vi "post-4616-1160681073.vi"(3 "New angle":dbl format="%.2f", 4 "Previous angle":dbl format="%.2f", 5 "Position % (50)":dbl=50.0 format="%.2f", 6 "Width":dbl format="%.2f") -> (0 "text orientation":T1(ring), 1 "Origin":cluster{dbl, dbl} {"?" format="%.2f"; "?" format="%.2f"})   [LabVIEW 2014]
doc: "This vi calculates the positions for the labels - and the orientation. Based on Origins for labels.vi in the NI example piechart.llb."
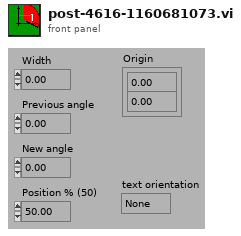
[diagram p1: front panel]
types:
  T1 = enum16{"None", "Stacked", "Clockwise", "Counterclockwise"}
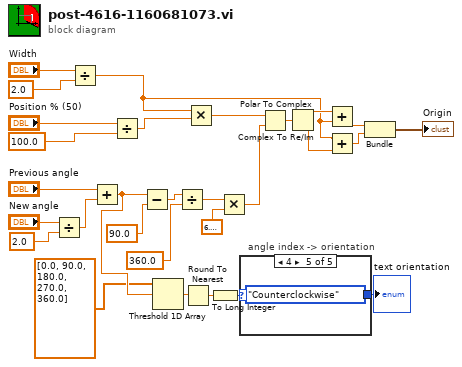
[diagram p0: block diagram]
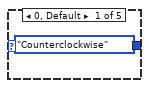
[diagram p2: hidden frame]
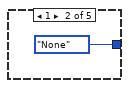
[diagram p3: hidden frame]
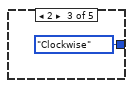
[diagram p4: hidden frame]
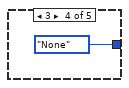
[diagram p5: hidden frame]
diagram:
  n1 = Divide(x="New angle", y=2.0) -> (x/y=w20:dbl)
  n2 = Divide(x="Width", y=2.0) -> (x/y=w14:dbl)
  n3 = Add(x="Previous angle", y=w20) -> (x+y=w6:dbl)
  n4 = Divide(x="Position % (50)", y=100.0) -> (x/y=w8:dbl)
  n5 = Subtract(x=w6, y=90.0) -> (x-y=w13:dbl)
  n6 = Threshold 1D Array(2:w6, 3:dbl[] [0.0, 90.0, 180.0, 270.0, 360.0] ("array of numbers or points")) -> (0:w4:dbl)  [unwired: 1 in]
  n7 = Divide(x=w13, y=360.0) -> (x/y=w17:dbl)
  n8 = Round To Nearest(number=w4) -> (nearest integer value=w3:dbl)
  n9 = Multiply(x=w14, y=w8) -> (x*y=w15:dbl)
  n10 = To Long Integer(number=w3) -> (32bit integer=w2:i32)
  n11 = Multiply(x=w17, y=6.283185307179586) -> (x*y=w22:dbl)
  n12 = case "angle index -> orientation" shown="4" w2 {
    tunnel: [T1."Counterclockwise" ("text orientation") T1."None" ("text orientation") T1."Clockwise" ("text orientation") T1."None" ("text orientation") T1."Counterclockwise" ("text orientation")] -> w1
    frame 0, Default {
    }
    frame 1 {
    }
    frame 2 {
    }
    frame 3 {
    }
    frame 4 {
    }
  }
  "text orientation" <- w1
  n13 = Polar To Complex(1:w22, 2:w15) -> (0:w21:cdb)
  n14 = Complex To Re/Im(x + iy=w21) -> (x=w24:dbl, y=w26:dbl)
  n15 = Add(x=w24, y=w14) -> (x+y=w27:dbl)
  n16 = Add(x=w14, y=w26) -> (x+y=w7:dbl)
  n17 = Bundle(w27, w7) -> (→"Origin":cluster{dbl, dbl})  [unwired: 1 in]
